vi "02.3 Messenger Channel.vi"() -> ()   [LabVIEW 2019]
uses:
  <vilib>/ChannelSupport/Channel Message/Read ID.vi
  <extravilib>/ChannelInstances/Stream-dbl/Endpoint.vi
  <extravilib>/ChannelInstances/Stream-dbl/EndpointRead.vi
  <extravilib>/ChannelInstances/Messenger-str/Wrapper.lvclass
  C:/Program Files/National Instruments/LabVIEW 2019/vi.lib/ChannelSupport/Channel Message/Channel Message.lvclass
  <extravilib>/ChannelInstances/Stream-dbl/Instantiate.vi
  <extravilib>/ChannelInstances/Stream-dbl/)Channel.vi
  <resource>/ChannelSupport/_ChannelSupport/WaitIfNeeded.vi
  <extravilib>/ChannelInstances/Messenger-str/Instantiate.vi
  <resource>/Channels/Messenger/Endpoint.vi
  <extravilib>/ChannelInstances/Messenger-str/Unwrap.vi
  <extravilib>/ChannelInstances/Messenger-str/Wrap.vi
  <extravilib>/ChannelInstances/Messenger-str.lvlib
  <extravilib>/ChannelInstances/Stream-dbl.lvlib
panel:
  out "Chart B":dbl(graph)
  out "Chart A":dbl(graph)
  in  "Stop 3":bool
  out "Chart":dbl(graph)
  out "Receiver 3":string
  out "Receiver 2":string
  in  "Stop 2":bool
  out "Receiver 1":string
  in  "Stop":bool
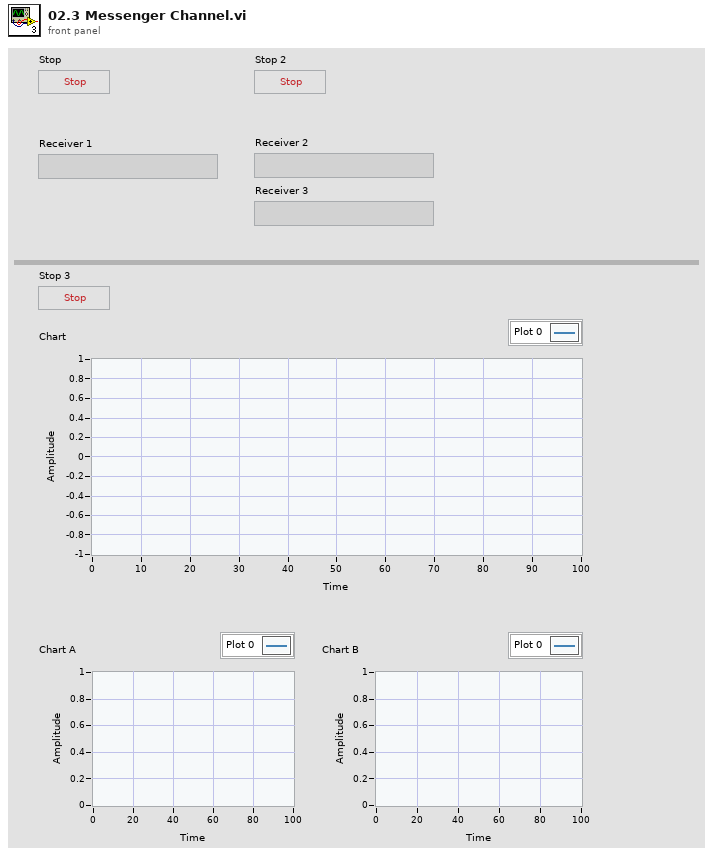
[diagram p1: front panel]
types:
  T1 = typedef "Stream-dbl.lvlib/)Channel.ctl" = refnum<queue>
  T2 = typedef "Messenger-str.lvlib/))Channel.ctl" = refnum<queue>
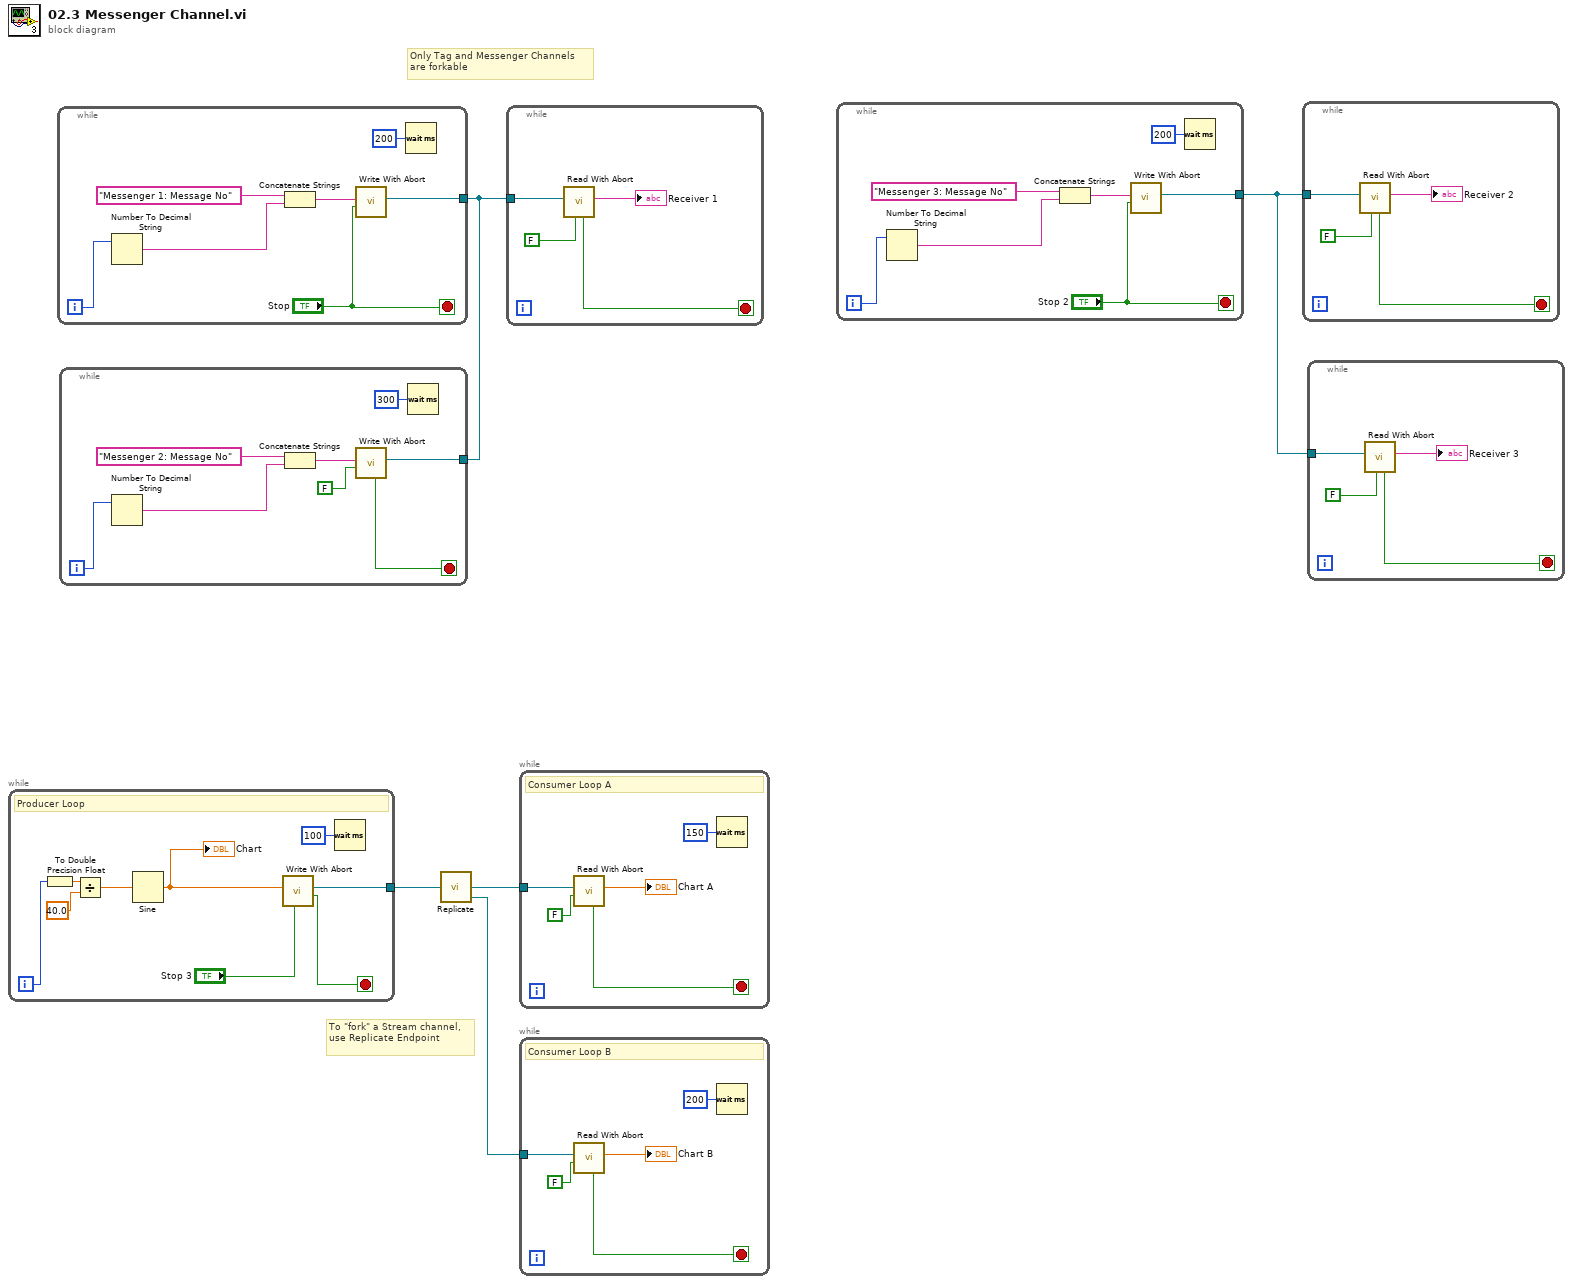
[diagram p0: block diagram]
diagram:
  # "To \"fork\" a Stream channel,\nuse Replicate Endpoint"
  # "Only Tag and Messenger Channels\nare forkable"
  n1 = while {
    tunnel: [w9] -> w3
    i -> [w12]
    stop <- w7 stop-if-true
    # "Producer Loop"
    n2 = To Double Precision Float(number=w12) -> (double precision float=w14:dbl)
    n3 = Divide(x=w14, y=40.0) -> (x/y=w13:dbl)
    n4 = Sine(x=w13) -> (sin(x)=w10:dbl)
    "Chart" <- w10
    n5 = call <resource>:"Write With Abort.vi"("abort"="Stop 3", "element"=w10) -> ("aborted?"=w7:bool, "channel"=w9:T1)  [unwired: 6 in, 2 out]
    n6 = Wait (ms)(milliseconds to wait=u32 100) -> ()  [unwired: 1 out]
  }
  n7 = while {
    tunnel: [w16] -> w5
    i -> [w21]
    stop <- "Stop" stop-if-true
    n8 = Number To Decimal String(number=w21) -> (decimal integer string=w20:string)  [unwired: 1 in]
    n9 = Concatenate Strings "Concatenate Strings"("Messenger 1: Message No" ("string"), w20) -> (w18:string)
    n10 = call <resource>:"Write With Abort.vi"("abort (F)"="Stop", "element"=w18) -> ("channel"=w16:T2)  [unwired: 6 in, 3 out]
    n11 = Wait (ms)(milliseconds to wait=u32 200) -> ()  [unwired: 1 out]
  }
  n12 = while {
    tunnel: w5 -> [w24]
    i -> [w29]
    stop <- w23 stop-if-true
    n13 = Number To Decimal String(number=w29) -> (decimal integer string=w28:string)  [unwired: 1 in]
    n14 = Concatenate Strings "Concatenate Strings"("Messenger 2: Message No" ("string"), w28) -> (w26:string)
    n15 = call <resource>:"Write With Abort.vi"("abort (F)"=FALSE, "element"=w26) -> ("channel"=w24:T2, "aborted?"=w23:bool)  [unwired: 6 in, 2 out]
    n16 = Wait (ms)(milliseconds to wait=u32 300) -> ()  [unwired: 1 out]
  }
  n17 = call <extravilib>:"Replicate.vi"("stream"=w3) -> ("stream copy 1"=w2:T1, "stream copy 2"=w1:T1)  [unwired: 7 in]
  n18 = while {
    tunnel: w5 -> [w33]
    stop <- w31 stop-if-true
    n19 = call <resource>:"Read With Abort.vi"("abort (F)"=FALSE, "channel"=w33) -> ("element"=→"Receiver 1":string, "aborted?"=w31:bool)  [unwired: 5 in, 3 out]
  }
  n20 = while {
    tunnel: w2 -> [w37]
    stop <- w35 stop-if-true
    # "Consumer Loop A"
    n21 = call <resource>:"Read With Abort.vi"("abort"=FALSE, "channel"=w37) -> ("element"=→"Chart A":dbl, "aborted?"=w35:bool)  [unwired: 4 in, 4 out]
    n22 = Wait (ms)(milliseconds to wait=u32 150) -> ()  [unwired: 1 out]
  }
  n23 = while {
    tunnel: w1 -> [w42]
    stop <- w40 stop-if-true
    # "Consumer Loop B"
    n24 = call <resource>:"Read With Abort.vi"("abort"=FALSE, "channel"=w42) -> ("element"=→"Chart B":dbl, "aborted?"=w40:bool)  [unwired: 4 in, 4 out]
    n25 = Wait (ms)(milliseconds to wait=u32 200) -> ()  [unwired: 1 out]
  }
  n26 = while {
    tunnel: [w45] -> w4
    i -> [w50]
    stop <- "Stop 2" stop-if-true
    n27 = Number To Decimal String(number=w50) -> (decimal integer string=w49:string)  [unwired: 1 in]
    n28 = Concatenate Strings "Concatenate Strings"("Messenger 3: Message No" ("string"), w49) -> (w47:string)
    n29 = call <resource>:"Write With Abort.vi"("abort (F)"="Stop 2", "element"=w47) -> ("channel"=w45:T2)  [unwired: 6 in, 3 out]
    n30 = Wait (ms)(milliseconds to wait=u32 200) -> ()  [unwired: 1 out]
  }
  n31 = while {
    tunnel: w4 -> [w54]
    stop <- w52 stop-if-true
    n32 = call <resource>:"Read With Abort.vi"("abort (F)"=FALSE, "channel"=w54) -> ("element"=→"Receiver 2":string, "aborted?"=w52:bool)  [unwired: 5 in, 3 out]
  }
  n33 = while {
    tunnel: w4 -> [w58]
    stop <- w56 stop-if-true
    n34 = call <resource>:"Read With Abort.vi"("abort (F)"=FALSE, "channel"=w58) -> ("element"=→"Receiver 3":string, "aborted?"=w56:bool)  [unwired: 5 in, 3 out]
  }
